vi "Turn to Angle.vi"(4 "Angle Tolerance":dbl=2.0, 5 "PID Gains":T1={"proportional gain (Kc)"=0.6, "integral time (Ti, min)"=0.0, "derivative time (Td, min)"=0.0} {"derivative time (Td, min)" format="%.3f"; "integral time (Ti, min)" format="%.3f"; "proportional gain (Kc)" format="%.3f"}, 6 "Rotation Multiplier":dbl, 7 "Target angle":dbl, 8 "Angle (radians; 0 = right)":dbl) -> (1 "Finished?":bool, 3 "Turn Set Point":dbl)   [LabVIEW 2015]
uses:
  <vilib>/addons/control/pid/pid.llb/PID Control Input Filter (DBL).vi
  <vilib>/addons/control/pid/pid.llb/PID (DBL).vi
  <vilib>/addons/control/pid/NI_PID_pid.lvlib
  Team900-VIs/Team900SwerveDrive/Team900SwerveDrive.lvlib
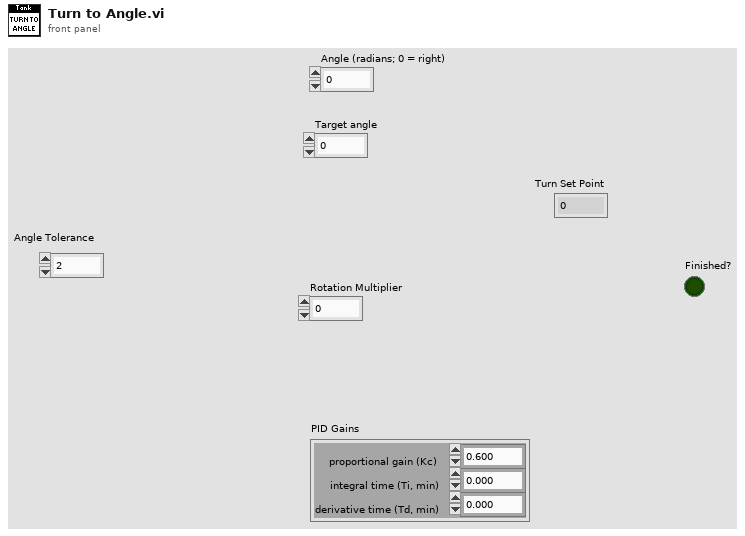
[diagram p1: front panel]
types:
  T1 = cluster{"proportional gain (Kc)":dbl, "integral time (Ti, min)":dbl, "derivative time (Td, min)":dbl}
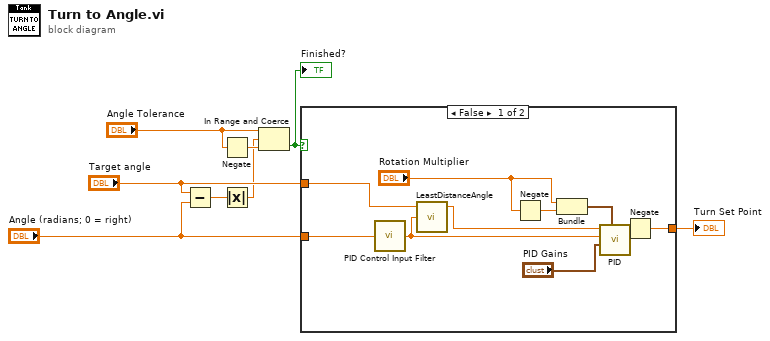
[diagram p0: block diagram]
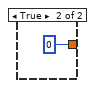
[diagram p2: hidden frame]
diagram:
  n1 = Subtract(x="Target angle", y="Angle (radians; 0 = right)") -> (x-y=w5:dbl)
  n2 = Negate(x="Angle Tolerance") -> (-x=w3:dbl)
  n3 = Absolute Value(x=w5) -> (abs(x)=w1:dbl)
  n4 = In Range and Coerce(upper limit="Angle Tolerance", x=w1, lower limit=w3) -> (In Range?=w2:bool)  [unwired: 1 out]
  "Finished?" <- w2
  n5 = case shown="False" w2 {
    tunnel: "Target angle" -> [w18 _]
    tunnel: [w9 0] -> w8
    tunnel: "Angle (radians; 0 = right)" -> [w16 _]
    frame False {
      n6 = call-poly <vilib>:"PID Control Input Filter.vi"("input"=w16) -> ("output"=w11:dbl)  [unwired: 4 in]
      n7 = call "LeastDistanceAngle.vi"("Current angle"=w11, "target angle (between pi and -pi) 2"=w18) -> ("output angle"=w10:dbl)  [unwired: 1 in, 2 out]
      n8 = Negate(x="Rotation Multiplier") -> (-x=w13:dbl)
      n9 = Bundle("Rotation Multiplier"="Rotation Multiplier", w13) -> (w12:cluster{"Rotation Multiplier":dbl, dbl})  [unwired: 1 in]
      n10 = call-poly <vilib>:"PID.vi"("output range"=w12, "PID gains"="PID Gains", "process variable"=w11, "setpoint"=w10) -> ("output"=w17:dbl)  [unwired: 6 in, 1 out]
      n11 = Negate(x=w17) -> (-x=w9:dbl)
    }
    frame True {
    }
  }
  "Turn Set Point" <- w8
